vi "Lifter Power Spectral Density of Gearbox.vi"() -> ()   [LabVIEW 2023]
doc: "This example shows the application of computing the cepstrum of a gearbox vibration signal to separate harmonic families in the power spectral density (PSD) of the signal.\n\nIn general, the PSD of a vibration signal that a gearbox generates consists of several families of harmonic peaks. These harmonic families are due to vibrations from different parts such as shafts and ball bearings, and each family of harmonic peaks belongs to a different part. It is difficult to separate harmonic families in the PSD directly. Cepstrum is an efficient tool you can use to separate different harmonic families. You can use these separated individual families in machine diagnosis.\n\nThis example removes a harmonic family from the PSD of an obtained vibration signal by completing the following steps:\n\n1) Compute the power cepstrum of the vibration signal from the gearbox. \n2) Use two cursors to select the fundamental peak of a harmonic family. All the peaks of the harmonic family will automatically be masked and removed from the power cepstrum. The resulting power cepstrum is called a liftered cepstrum.\n3) Reconstruct the PSD from the liftered cepstrum with the TSA Lifter PSD VI. The reconstructed PSD shows that the selected harmonic family has been removed.\n\nThis example uses the TSA Lifter PSD VI to remove a harmonic family from the PSD of a gearbox signal.\n\n<b>Instructions:</b>\n1) Run this VI.\n2) Move the cursors to specify the location range of the fundamental peak.\n3) Observe the liftered power spectrum."
uses:
  <vilib>/addons/_Advanced Signal Processing/NI_AdvSigProcTSA.lvlib
panel:
  in  "stop":bool
  out "Power Cepstrum of the Gearbox Vibration Signal":cluster{"t0":dbl, "dt":dbl, "mask":dbl[]}[](graph)
  out "PSD of the Gearbox Vibration Signal":cluster{"f0":dbl, "df":dbl, "S(f)":dbl[]}[](graph)
  # "Overview: Shows the application of computing the cepstrum of a gearbox vibration signal to separate harmonic families in the power spectral density (PSD) of the signal.\nRequirements: LabVIEW Full Development System, Advanced Signal Processing Toolkit\nInstructions: \n1. Run this VI.\n2. Move the cursors to specify the location range of the fundamental peak.\n3. Observe the liftered power spectrum.\n4. Click Stop to stop the VI."
  # "Move the cursors to specify the location of the fundamental peak."
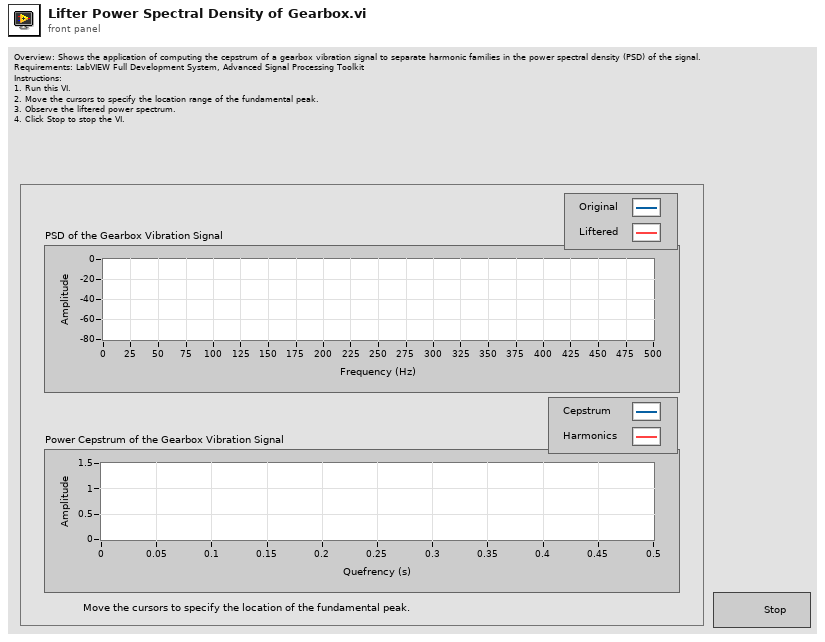
[diagram p1: front panel]
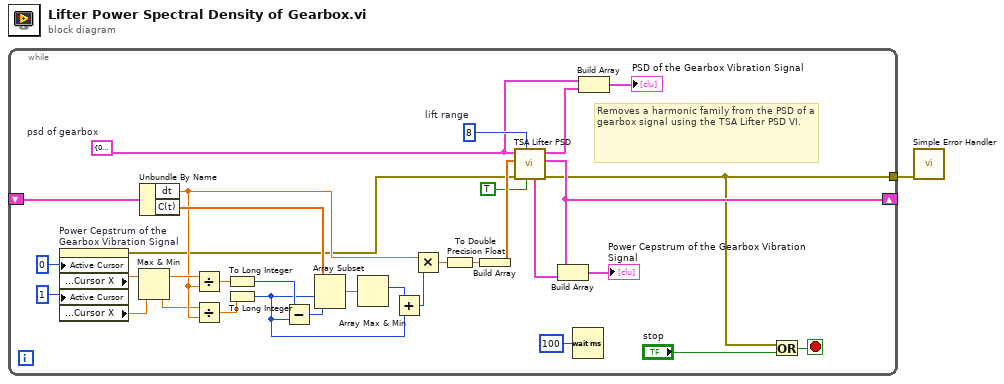
[diagram p0: block diagram]
diagram:
  n1 = while {
    shift-right: [w14] -> _
    shift-left: _ -> [w17]
    tunnel: [w3] -> w1
    stop <- w4 stop-if-true
    w33 = 8  # lift range
    w26 = cluster{dbl, dbl, "magnitude":dbl[]} {0.0, 1.0, "magnitude"=[-65.08349763453558, -64.65753158949333, -67.69363425301734, -66.50111220211801, -64.64011031741015, -62.03979454459139, -58.47674081794985, -57.56095323578968, -57.786497026776914, -56.70644229457807, -53.792026682888554, -51.839017674611924, -54.76390983871177, -50.28363551857475, -47.26453777368984, -44.07128490861723, -35.7239993536833, -34.63271643581042, -43.35647844599719, -46.89120817643429, -49.653589174786354, -49.795700279175456, -50.81554113239497, -52.20827080797974, -51.3035791056151, -50.95692843981261, -49.652141198804955, -49.54665593133544, -47.336142471967584, -47.26975663240669, -45.065944616571514, -44.48137206225204, -37.9808504739474, -29.38239917025544, -31.52797059173235, -42.394448388600516, -42.8012051081507, -43.507844254742224, -44.2712262425302, -44.591671597698706, -44.69142481318143, -44.480742512919775, -43.64557926394739, -41.83519997418033, -41.31976338830924, -41.5013165945771, -40.47218022726922, -39.662618524456875, -39.76184594975717, -35.59320467102832, -32.903597822689605, -37.386735326936616, -38.978676450949415, -41.91783340043604, -43.47478289837662, -42.08229180090696, -39.601132327588445, -38.99830565909317, -40.15980062501029, -39.66064884360311, -39.29688895188826, -37.917598697118684, -39.74113343047902, -38.83008472796174, -38.44084622658349, -37.44582264666603, -32.391149377837856, -31.92623665923406, -37.48112025042427, -37.364250099755715, -37.34202695813699, -38.6957479922975, -37.414247485509414, -36.79440574222323, -37.4290366507549, -36.469295161838915, -35.85278151923913, -36.583337115731595, -35.64719569883153, -33.920788956396734, -31.04196325875513, -29.18181816136336, -27.082682997511334, -23.969986741215394, -25.519363701869953, -26.34443129197755, -28.307955492942853, -31.067754501235825, -29.765896377549097, -28.6947246979041, -29.09596268503643, -31.80275392024377, -31.369742969096833, -28.22115472258059, -28.555320612572114, -30.096963400910187, -29.269172627147178, -28.606109214551093, -26.68344260769446, -22.894117275430492, -18.56522318324473, -23.369423364955498, -25.29647699268601, -24.8605919982989, -26.289808896155424, -28.92288744382684, -28.483310380590247, -28.42675577544501, -27.91622077074338, -28.765045088614322, -26.06337423424341, -25.34984811198705, -25.652951928718586, -25.860847685493052, -25.404827350926023, -24.671183413401074, -18.843155002014576, -17.368218530851106, -23.252083555996293, -24.112745523008556, -25.387773479654626, -26.80030398716308, -27.530752570658173, -27.70137070971529, -27.600110477136756, -27.272511543837716, -26.55656066902393, -26.432493571625507, -26.029824938444456, -26.159542231255056, -26.522407542043048, -25.21102354926162, -22.80232643869943, -18.256734639546615, -19.974572334673372, -23.826110953245134, -22.52838311003468, -24.58774667721964, -25.72226014504826, -25.897865176856385, -26.48924203274153, -27.792464381504477, -27.42609978034446, -26.586866509115673, -26.139606220517738, -26.24514996036702, -25.40332689304688, -24.55051554138421, -24.87310552060917, -20.659074337398412, -17.237085924070932, -21.793501975901272, -25.720133315062952, -25.466356673330015, -25.53325951019427, -25.758069155454454, -26.80999214760938, -28.013158624252455, -27.076385302661905, -26.976079954886135, -27.232368622110798, -27.89314028800581, -27.701070519940107, -28.0438075970767, -27.825409799781823, -26.313895592620575, -23.643771308690305, -23.522915319132732, -26.703946741827373, -26.781602344639296, -26.348986691834163, -26.541482974645124, -27.139002170411743, -27.543898881826433, -28.48193405127262, -28.826894531385044, -28.329333017596223, -29.063378837258046, -29.854581909095337, -29.6194619576679, -27.609234727000626, -28.02420967371793, -26.548996611942634, -21.07869793654581, -23.403809816103944, -28.214459804097114, -28.74293403739593, -28.51245484339506, -29.00685484886398, -29.45511450729561, -29.22220256666101, -29.34930522238275, -31.36558510184097, -31.1531082455406, -30.34708852382915, -29.875019332453284, -29.141001191051423, -28.82227352960459, -28.86992462817574, -27.138685474418132, -23.50681690387511, -27.009848355720735, -30.39646061056597, -30.391347908902024, -30.608979770743492, -31.203660185646935, -30.841431665416238, -31.85409993700237, -31.983609577536924, -31.821100025398334, -31.928686255788413, -31.476736894977087, -31.355610453487373, -29.996934250709693, -29.8179167870286, -28.64580627621968, -23.355530031703537, -22.332003128553627, -28.914245807995673, -31.86998595880798, -32.72371376127404, -33.93039230747832, -32.46431646835838, -32.04802055164055, -33.08538227478093, -34.20562497018763, -34.103054323432154, -33.97765763012817, -33.771252192980114, -33.34555837255314, -32.680790613481655, -33.57408261566745, -32.153918009307645, -29.28494464972303, -29.81805352784299, -31.404800878364835, -33.79895907060019, -34.4629921510231, -34.08492446335022, -34.837205865599536, -35.90235775682231, -35.45310638343069, -36.19582572858239, -36.40922350174688, -36.10792244416743, -36.55205205203416, -36.813365745614604, -34.23707542799687, -34.02206730053781, -32.17545757323646, -29.62493439347691, -33.530608636109534, -35.53723397153916, -36.4810066920277, -36.58937174553193, -36.24006741122547, -37.04850239747388, -36.70507766732527, -38.33331922723585, -38.730651752217376, -37.54007399685374, -37.239044549947515, -37.40497595697646, -35.97328111491131, -36.47404191091287, -37.999615807064295, -35.800956544485885, -35.27626287936688, -36.994913751786626, -37.39516447516658, -37.87271870801962, -37.8771925888558, -37.40142070785039, -38.94625015726809, -38.91534210520138, -38.99317260054029, -40.627607945975306, -40.66620006653132, -40.32928183543687, -40.76024274768058, -38.772717890837576, -38.144679904425324, -37.21041413453159, -36.548519271597485, -38.36966032131208, -38.74030523581907, -38.155908843178615, -38.932616298924245, -41.497646730917566, -41.573790987913235, -40.5026300728441, -40.875501510045126, -43.7355562672568, -41.30169208944867, -42.74394070976089, -42.77992660976419, -40.5711696372538, -40.05286860441943, -42.851168424701285, -39.43542310997345, -36.281180307314955, -38.01914903580149, -40.40617148647112, -40.50860225029144, -40.7274022412668, -41.808571203885414, -42.15949434976062, -42.73997731037887, -43.27430125816663, -43.52370398462217, -43.55803216506027, -42.91899732060828, -43.6959836256941, -45.29892689043723, -46.27921387306835, -44.233507366941, -42.37934791270112, -41.742307069593096, -41.814368640377324, -43.73029808129804, -44.24560928702473, -46.470799892531495, -44.803696112460294, -45.08544108499092, -44.60131813800754, -47.167192630225315, -47.57136015332314, -47.141017404574406, -46.900254950680434, -45.9241022672347, -43.7942100479124, -45.948520132980065, -45.656952448237725, -44.27700014572107, -44.364302300685424, -44.27838394777568, -45.61044700266291, -46.87254029127034, -46.82605166407376, -47.49027315641637, -47.28992888717027, -47.65968883528203, -48.00402333953735, -47.19874622460436, -47.21835876990937, -49.516191194689945, -48.087073880384, -47.248190379066514, -48.9636347667339, -47.86016321508208, -46.399889890153226, -48.00986630323777, -47.9501500352091, -47.19983009028347, -49.55239562675501, -48.455212586986356, -47.610734643643504, -48.83967333369079, -49.43908791547515, -50.2386749621771, -49.66887014197577, -49.213825800358165, -49.688260528191634, -46.53904831306412, -47.38995468036363, -48.84531007378744, -49.142844784672796, -48.20407872660887, -49.676070973803625, -50.34452456403169, -49.424659902853364, -51.78100955381447, -51.55034393825676, -50.91978458838244, -51.42357830771839, -50.93749536141627, -51.65906950214119, -54.37957570131146, -52.661357384976164, -51.79503334868617, -51.73703062558552, -51.59601002821337, -49.93862838805125, -48.96469821170926, -49.52401592275463, -50.52054548359315, -50.19347078834761, -52.05648426789853, -51.166802188913856, -48.29513277407116, -50.81448288210849, -51.80919387350943, -54.08787725968906, -54.029717105190294, -53.99695866895661, -52.42611337573365, -54.19340565658233, -53.387084852487774, -52.93142137166886, -52.673064770095735, -52.746361013827034, -53.35559447192792, -54.20138601936786, -52.77271154024977, -55.11951893999004, -53.84836113612364, -53.437914335183414, -53.85904720024403, -53.30027583740102, -54.291759647764465, -54.79500615162989, -54.69172713325926, -55.32598301923622, -53.75775878764567, -55.22549868357126, -54.26169911698211, -52.327122796764066, -53.256141326363284, -53.98693488782898, -53.715784315497345, -54.029080510252044, -55.305973597169675, -52.724696594474636, -52.59709623007157, -55.034876663057055, -56.60592407395902, -57.1227526195879, -55.43311090982836, -55.87498219391529, -56.52651904785116, -56.40746138904621, -56.15743418641166, -54.8219550512366, -54.32041219394348, -55.59324073762305, -56.57155533833937, -54.47908745696522, -55.6503927630432, -57.46220012056768, -55.71627205069524, -55.5026459715678, -56.17183006340957, -58.21077015972009, -57.58281858076394, -57.71366651609047, -58.74638135350821, -56.702155117398014, -56.88140788560123, -58.660052789557696, -57.03057761580151, -59.348913738869314, -58.07130143983738, -59.32721146371812, -57.4081350490226, -59.56035089961272, -59.92568918736731, -57.76987607408423, -58.65323568018481, -58.042764780246, -59.027809963455724, -59.35574496250108, -60.02178527558877, -60.43324461364074, -58.614062160847325, -58.566498225303015, -60.24406662070122, -60.79501554288793, -61.60709655443958, -60.18959193912184, -60.0982502092313, -60.27142631084706, -61.13013387851021, -62.406821074744215, -61.48556863754862, -60.44357515771936, -61.9982260707609, -63.397523892314844, -62.23300319131829, -63.106606456545066, -60.39096613533658, -60.79267545880779, -62.822906004637574, -62.17459068337344, -64.14115857546899, -63.476620241575425, -63.80850511585331, -62.71851780026382, -63.03806701041773, -63.468269245586356, -63.7455327246991, -63.92582827134081, -63.74043111879029, -63.48274318263854, -65.14946998705464, -63.328587978410475, -63.26524825802909, -63.07451619013604, -63.30061647499452, -64.30076505937369, -64.05068373018855]}  # psd of gearbox
    # "Removes a harmonic family from the PSD of a gearbox signal using the TSA Lifter PSD VI."
    n2 = property on="Power Cepstrum of the Gearbox Vibration Signal" class="WFGraph (strict)"("Active Cursor"=u32 0, "Active Cursor"=u32 1) -> (error out=w6:errorcluster, "Cursor.Cursor Position:Cursor X"=w28:dbl, "Cursor.Cursor Position:Cursor X"=w27:dbl)  [unwired: 2 in, 1 out]
    n3 = Max & Min(x=w28, y=w27) -> (max(x,y)=w25:dbl, min(x,y)=w8:dbl)
    n4 = Unbundle By Name(w17) -> ("dt"=w9:dbl, "C(t)"=w16:dbl[])
    n5 = Divide(x=w25, y=w9) -> (x/y=w11:dbl)
    n6 = Divide(x=w8, y=w9) -> (x/y=w10:dbl)
    n7 = To Long Integer(number=w11) -> (32bit integer=w22:i32)
    n8 = To Long Integer(number=w10) -> (32bit integer=w20:i32)
    n9 = Subtract(x=w22, y=w20) -> (x-y=w24:i32)
    n10 = Array Subset(array=w16, index=w20, length=w24) -> (w23:dbl[])
    n11 = Array Max & Min(array=w23) -> (max index (indices)=w21:i32)  [unwired: 3 out]
    n12 = Add(x=w21, y=w20) -> (x+y=w13:i32)
    n13 = Multiply(x=w9, y=w13) -> (x*y=w12:dbl)
    n14 = To Double Precision Float(number=w12) -> (double precision float=w19:dbl)
    n15 = Build Array(w19) -> (w18:dbl[])
    n16 = call <vilib>:"TSA Lifter PSD.vi"("dB on? (T)"=TRUE ("dB On? (T)"), "lifter range"=w33, "error in (no error)"=w6, "base t"=w18, "PSD"=w26) -> ("error out"=w3:errorcluster, "power cepstrum"=w14:cluster{"t0":dbl, "dt":dbl, "C(t)":dbl[]}, "liftered PSD"=w31:cluster{"f0":dbl, "df":dbl, "S(f)":dbl[]}, "liftering mask"=w15:cluster{"t0":dbl, "dt":dbl, "mask":dbl[]})  [unwired: 3 out]
    n17 = Build Array(w14, w15) -> (→"Power Cepstrum of the Gearbox Vibration Signal":cluster{"t0":dbl, "dt":dbl, "mask":dbl[]}[])
    n18 = Wait (ms)(milliseconds to wait=u32 100) -> ()  [unwired: 1 out]
    n19 = Build Array(w26, w31) -> (→"PSD of the Gearbox Vibration Signal":cluster{"f0":dbl, "df":dbl, "S(f)":dbl[]}[])
    n20 = Or(x=w3, y="stop") -> (x .or. y?=w4:bool)
  }
  n21 = call <vilib>:"Simple Error Handler.vi"("error in (no error)"=w1) -> ()  [unwired: 4 in, 5 out]
